vi "Get Cycles.vi"(8 "error in (no error)":errorcluster, 11 "Attributes in":refnum<class "Attributes.lvclass">) -> (0 "error out":errorcluster, 3 "Attributes out":refnum<class "Attributes.lvclass">)   [LabVIEW 2021, in "Attributes.lvclass"]
uses:
  Attributes.lvclass
  Attributes.lvclass/Attributes.ctl
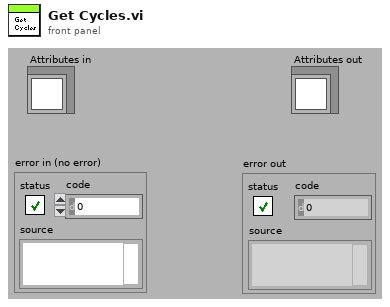
[diagram p1: front panel]
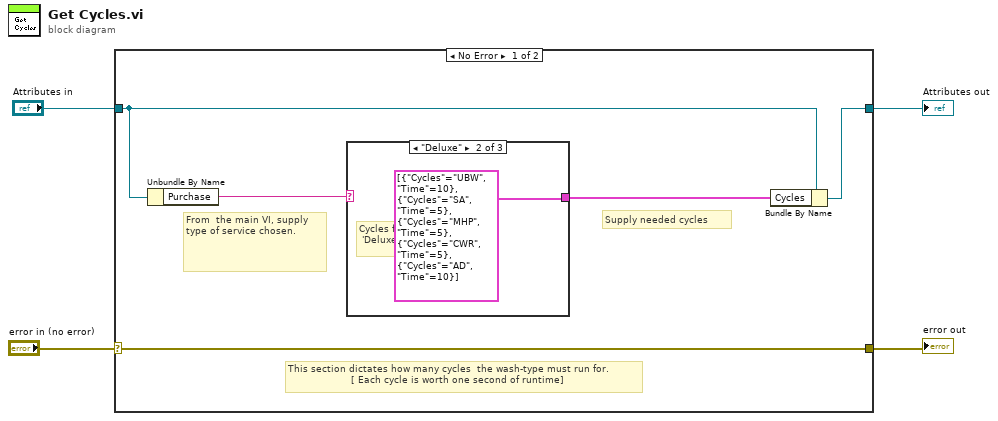
[diagram p0: block diagram]
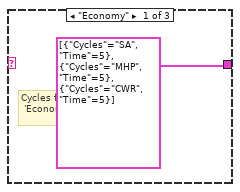
[diagram p2: hidden frame]
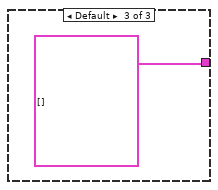
[diagram p3: hidden frame]
diagram:
  n1 = case shown="No Error" "error in (no error)" {
    selector: "error in (no error)" -> [w9 w14]
    tunnel: [w9 w14] -> w3
    tunnel: [w6 w13] -> w1
    tunnel: "Attributes in" -> [w7 w13]
    frame No Error {
      # "Supply needed cycles"
      # "From  the main VI, supply type of service chosen."
      # "This section dictates how many cycles  the wash-type must run for.\n                     [ Each cycle is worth one second of runtime]"
      n2 = Unbundle By Name(w7) -> ("Purchase"=w8:string)
      n3 = case shown="\"Deluxe\"" w8 {
        tunnel: [cluster{"Cycles":string, "Time":u32}[] [{"Cycles"="SA", "Time"=5}, {"Cycles"="MHP", "Time"=5}, {"Cycles"="CWR", "Time"=5}] ("Cycles") cluster{"Cycles":string, "Time":u32}[] [{"Cycles"="UBW", "Time"=10}, {"Cycles"="SA", "Time"=5}, {"Cycles"="MHP", "Time"=5}, {"Cycles"="CWR", "Time"=5}, {"Cycles"="AD", "Time"=10}] ("Cycles") cluster{"Cycles":string, "Time":u32}[] [] ("Cycles")] -> w5
        frame "Economy" {
          # "Cycles for\n 'Economy'"
        }
        frame "Deluxe" {
          # "Cycles for\n 'Deluxe'"
        }
        frame Default {
        }
      }
      n4 = Bundle By Name(cluster=w7, "Cycles"=w5) -> (w6:refnum<class "Attributes.lvclass">)
    }
    frame Error {
    }
  }
  "error out" <- w3
  "Attributes out" <- w1
